vi "Validate Disconnection.vi"(8 "error in (no error)":errorcluster, 9 "channel 2":string, 10 "channel 1":string, 11 "SLSC Switch in":refnum<class "SLSC Switch.lvclass">) -> (0 "error out":errorcluster, 3 "SLSC Switch out":refnum<class "SLSC Switch.lvclass">)   [LabVIEW 2016, in "SLSC Switch.lvlib" / "SLSC Switch.lvclass"]
uses:
  SLSC Switch.lvclass
  SLSC Switch.lvclass/SLSC Switch.ctl
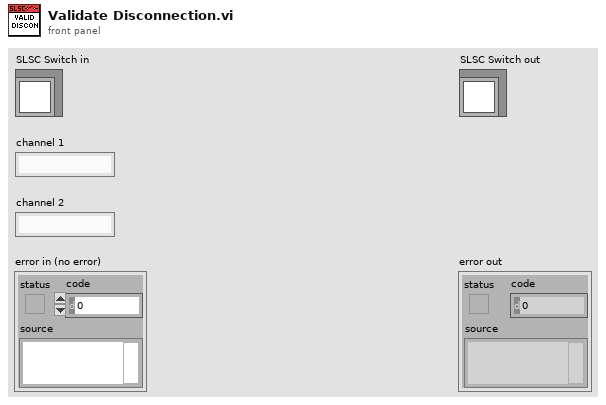
[diagram p1: front panel]
types:
  T1 = typedef "SLSC Switch.lvlib/SLSC Switch.lvclass/Connection.ctl" = cluster{"channel 1":string, "channel 2":string}
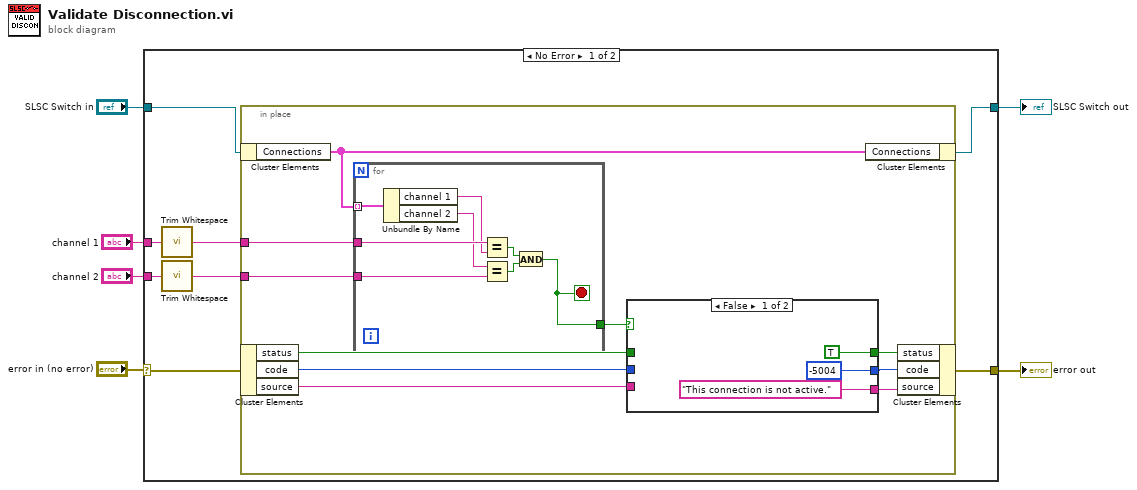
[diagram p0: block diagram]
diagram:
  n1 = case shown="No Error" "error in (no error)" {
    selector: "error in (no error)" -> [w9 w40]
    tunnel: [w8 w40] -> w1
    tunnel: [w14 w39] -> w2
    tunnel: "channel 1" -> [w13 _]
    tunnel: "channel 2" -> [w12 _]
    tunnel: "SLSC Switch in" -> [w7 w39]
    frame No Error {
      n2 = call <vilib>:"Trim Whitespace.vi"("string"=w13) -> ("trimmed string"=w11:string)  [unwired: 1 in]
      n3 = call <vilib>:"Trim Whitespace.vi"("string"=w12) -> ("trimmed string"=w10:string)  [unwired: 1 in]
      n4 = in-place {
        in-place-border: w11 -> [w24]
        in-place-border: w10 -> [w23]
        n5 = in-place-cluster #1(w7) -> ("Connections"=w22:T1[])
        n6 = in-place-cluster #2(w9) -> ("status"=w19:bool, "code"=w18:i32, "source"=w17:string)
        n7 = for {
          tunnel: w22 -> [w38] mode=indexing
          tunnel: w24 -> [w37]
          tunnel: w23 -> [w34]
          tunnel: [w31] -> w21
          stop <- w31 stop-if-true
          n8 = Unbundle By Name(w38) -> ("channel 1"=w36:string, "channel 2"=w35:string)
          n9 = Equal?(x=w37, y=w36) -> (x = y?=w33:bool)
          n10 = Equal?(x=w35, y=w34) -> (x = y?=w32:bool)
          n11 = And(x=w33, y=w32) -> (x .and. y?=w31:bool)
        }
        n12 = case shown="False" w21 {
          tunnel: ["This connection is not active." ("source") w28] -> w15
          tunnel: [-5004 ("code") w29] -> w16
          tunnel: [TRUE w30] -> w20
          tunnel: w19 -> [_ w30]
          tunnel: w18 -> [_ w29]
          tunnel: w17 -> [_ w28]
          frame False {
          }
          frame True {
          }
        }
        n13 = in-place-cluster #1("Connections"=w22) -> (w14:refnum<class "SLSC Switch.lvclass">)
        n14 = in-place-cluster #2("status"=w20, "code"=w16, "source"=w15) -> (w8:errorcluster)
      }
    }
    frame Error {
    }
  }
  "error out" <- w1
  "SLSC Switch out" <- w2
